vi "Statically-sized Cluster Array.vi"   [LabVIEW 2020, in "Memory Manager Tests.lvlib" / "Malleable Type Tests.lvclass"]
uses:
  Malleable Type Tests.lvclass
  dfef2f2c-28b0-4c73-9b6c-043406a820fb.vi
  Source/Classes/Pointer/Check Null Pointer.vi
  Source/Classes/Pointer/Get Size.vi
  Source/Classes/Pointer/Get Address.vi
  Source/Classes/Pointer/Errors.vi
  Source/Classes/Pointer/Out of Bounds.vi
  Source/Classes/Pointer/Pointer.lvclass
  Malleable Type Tests.lvclass/Malleable Type Tests.ctl
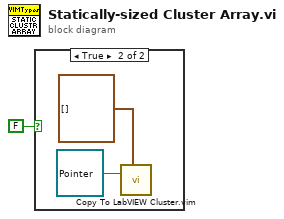
[diagram p0: block diagram]
diagram:
  n1 = case shown="True" FALSE {
    frame False {
    }
    frame True {
      n2 = call "Copy To LabVIEW Cluster.vim"("Type"=cluster{i32, i32, i32}[] [], "Pointer in"=refnum<class "Pointer.lvclass"> refnum) -> ()  [unwired: 7 in, 3 out]
    }
  }
